vi "TPNT_GetTP2Str.vi"(7 "device":string, 10 "TPs":T1[](array[typedef]) {"Log"."updaterate" format="%.2f"; "Samples"."Values" format="%.2f"; "Samples"."samples" min=1 step=1; "Limits"."Nominal" format="%.2f"; "Limits"."Upper" format="%.2f"; "Limits"."Lower" format="%.2f"; "update_rate" format="%.2f"}) -> (2 "String":string)   [LabVIEW 2016]
uses:
  TPNT_TP.ctl
  TPNT_Limits.ctl
  TPNT_Samples.ctl
  TPNT_Log.ctl
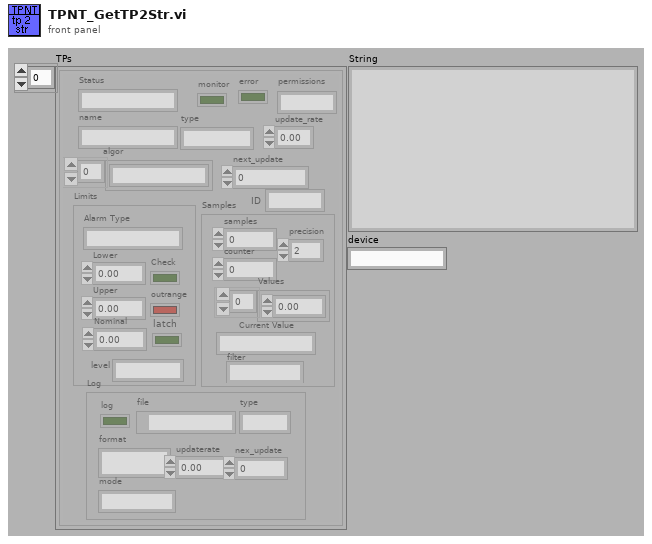
[diagram p1: front panel]
types:
  T1 = typedef "TPNT_TP.ctl" = cluster{"name":string, "type":string, "algor":string[], "update_rate":sgl, "Limits":T2, "Samples":T3, "next_update":u32, "Status":string, "monitor":bool, "error":bool, "Log":T4, "permissions":string, "ID":string}
  T2 = typedef "TPNT_Limits.ctl" = cluster{"Alarm Type":string, "Lower ":dbl, "Upper":dbl, "Nominal":dbl, "outrange":bool, "Check":bool, "latch":bool, "level":string}
  T3 = typedef "TPNT_Samples.ctl" = cluster{"samples":i32, "counter":i32, "Values":dbl[], "Current Value":string, "filter":string, "precision":u8}
  T4 = typedef "TPNT_Log.ctl" = cluster{"log":bool, "file":path, "type":string, "format":string, "updaterate":dbl, "nex_update":u32, "mode":string}
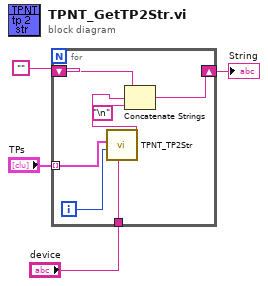
[diagram p0: block diagram]
diagram:
  n1 = for {
    tunnel: "TPs" -> [w8] mode=indexing
    shift-right: [w11] -> w2
    shift-left: "" -> [w7]
    tunnel: "device" -> [w5]
    i -> [w6]
    n2 = call "TPNT_TP2Str.vi"("device"=w5, "index in"=w6, "TestPoint In"=w8) -> ("TP out"=w10:string)  [unwired: 8 out]
    n3 = Concatenate Strings(w7, w10, "\n") -> (w11:string)
  }
  "String" <- w2
